vi "Read Module Decimation.vi"(7 "Module ID":string, 8 "error in":errorcluster, 11 "Standard Engine Repo Data in":refnum<class "Standard Engine Configuration.lvclass">) -> (0 "error out":errorcluster, 2 "Module Decimation":T1={"Decimation"=1, "Offset"=0, "sort order"=0, "async?"=FALSE}, 3 "Standard Engine Repo Data out":refnum<class "Standard Engine Configuration.lvclass">)   [LabVIEW 2013, in "Standard Engine Configuration.lvclass"]
doc: "Returns the decimation values for the specified module that were configured using the 'Write Module Decimation.vi'."
uses:
  Standard Engine Configuration.lvclass
  Module Decimation.ctl
  Standard Engine Configuration.lvclass/Standard Engine Configuration.ctl
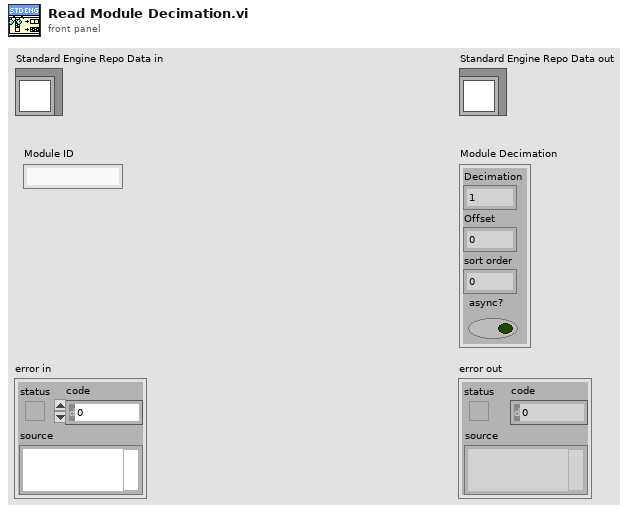
[diagram p1: front panel]
types:
  T1 = typedef "Standard Engine Configuration.lvclass/Module Decimation.ctl" = cluster{"Decimation":u16, "Offset":u16, "sort order":i32, "async?":bool}
  T2 = typedef "Standard Engine Configuration.lvclass/Module Specific Configuration.ctl" = cluster{"Module ID":string, "Module Decimation":T1, "error tag":string, "error responses":T3}
  T3 = typedef "Standard Engine Configuration.lvclass/error responses.ctl" = cluster{"unknown":T4, "trivial":T4, "critical":T4, "recoverable":T4}
  T4 = typedef "Standard Engine Configuration.lvclass/error options.ctl" = cluster{"clear":bool, "notify":bool, "remove module":bool, "abort engine":bool, "go to safe state":bool, "recover module":bool}
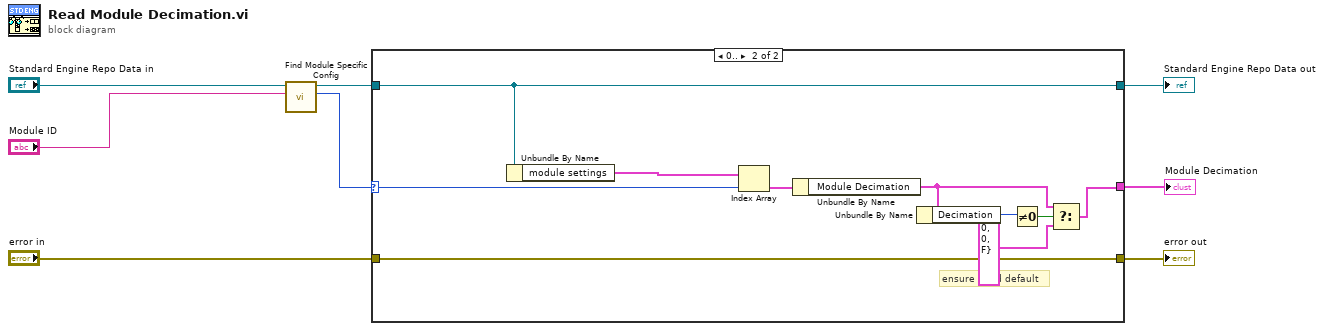
[diagram p0: block diagram]
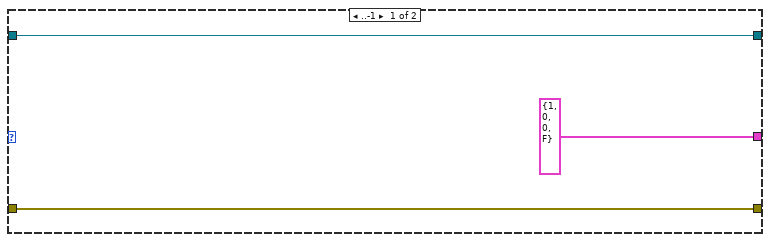
[diagram p2: hidden frame]
diagram:
  n1 = call "Find Module Specific Config.vi"("Module ID"="Module ID", "Standard Engine Repo Data in"="Standard Engine Repo Data in") -> ("Index"=w1:i32, "Standard Engine Repo Data out"=w2:refnum<class "Standard Engine Configuration.lvclass">)  [unwired: 8 in]
  n2 = case shown="0.." w1 {
    selector: w1 -> [_ w18]
    tunnel: w2 -> [w11 w19]
    tunnel: [T1 {"Decimation"=1, "Offset"=0, "sort order"=0, "async?"=FALSE} ("Module Decimation") w13] -> w5
    tunnel: "error in" -> [w10 w17]
    tunnel: [w10 w17] -> w3
    tunnel: [w11 w19] -> w6
    frame ..-1 {
    }
    frame 0.. {
      # "ensure good default"
      n3 = Unbundle By Name(w19) -> ("module settings"=w21:T2[])
      n4 = Index Array(array=w21, index=w18) -> (element=w20:T2)
      n5 = Unbundle By Name(w20) -> ("Module Decimation"=w14:T1)
      n6 = Unbundle By Name(w14) -> ("Decimation"=w16:u16)
      n7 = Not Equal To 0?(x=w16) -> (x != 0?=w15:bool)
      n8 = Select(t=w14, s=w15, f=T1 {"Decimation"=1, "Offset"=0, "sort order"=0, "async?"=FALSE} ("Module Decimation")) -> (s? t:f=w13:T1)
    }
  }
  "error out" <- w3
  "Standard Engine Repo Data out" <- w6
  "Module Decimation" <- w5
